vi "Read Reference phase.vi"(8 "error in (no error)":errorcluster, 11 "Lock-in Detector in":refnum<class "Lock-in Detector.lvclass">) -> (0 "error out":errorcluster, 2 "Reference phase":dbl, 3 "Lock-in Detector out":refnum<class "Lock-in Detector.lvclass">)   [LabVIEW 2020, in "Lock-in Detector.lvclass"]
uses:
  Lock-in Detector.lvclass
  Lock-in Detector.lvclass/Lock-in Detector.ctl
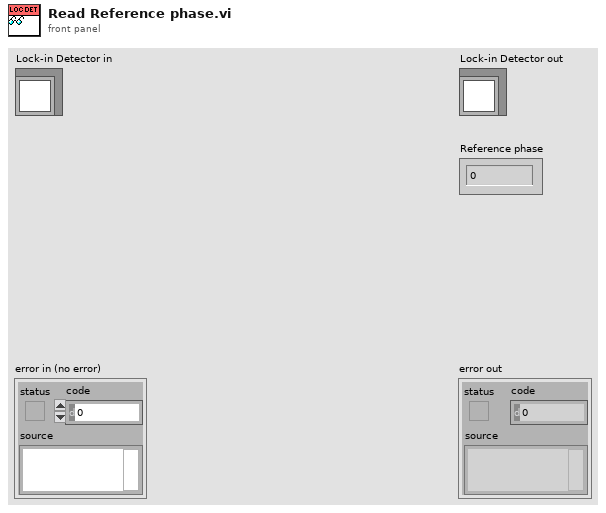
[diagram p1: front panel]
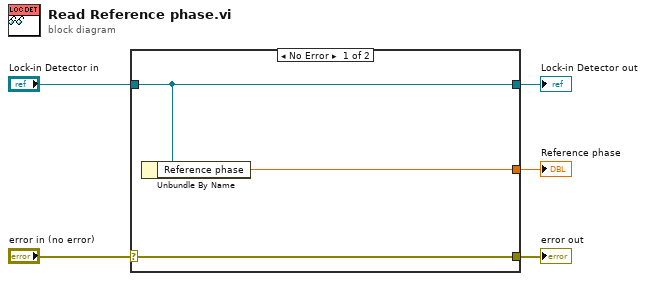
[diagram p0: block diagram]
diagram:
  n1 = case shown="No Error" "error in (no error)" {
    selector: "error in (no error)" -> [w8 w9]
    tunnel: [w8 w9] -> w4
    tunnel: [w7 w10] -> w2
    tunnel: "Lock-in Detector in" -> [w7 w10]
    tunnel: [w6 _] -> w1
    frame No Error {
      n2 = Unbundle By Name(w7) -> ("Reference phase"=w6:dbl)
    }
    frame Error {
    }
  }
  "error out" <- w4
  "Lock-in Detector out" <- w2
  "Reference phase" <- w1
